vi "Phasor Convert Ratio to Amplitude Ratio & Average Lifetime.vi"(6 "Compute Amplitude Ratio":bool, 8 "error in (no error)":errorcluster, 9 "Reference Lifetime 2":dbl[unit], 10 "Reference Lifetime 1":dbl[unit], 11 "Phasor Ratio (f1)":dbl) -> (0 "error out":errorcluster, 1 "Average Lifetime":dbl[unit], 3 "Phasor/Amplitude Ratio":dbl, 4 "Average Lifetime Caption":string, 5 "Phasor Ratio Plot Name Suffix":string)   [LabVIEW 2021, in "Phasor.lvlib"]
uses:
  Phasor.lvlib
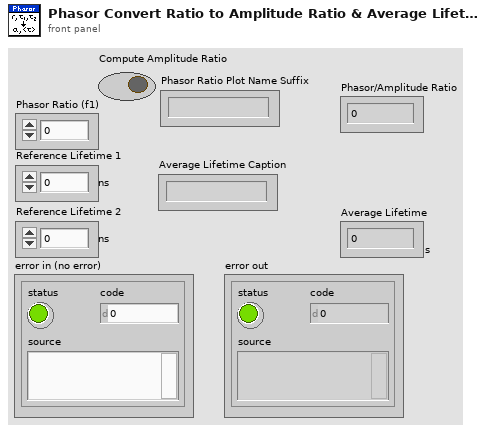
[diagram p1: front panel]
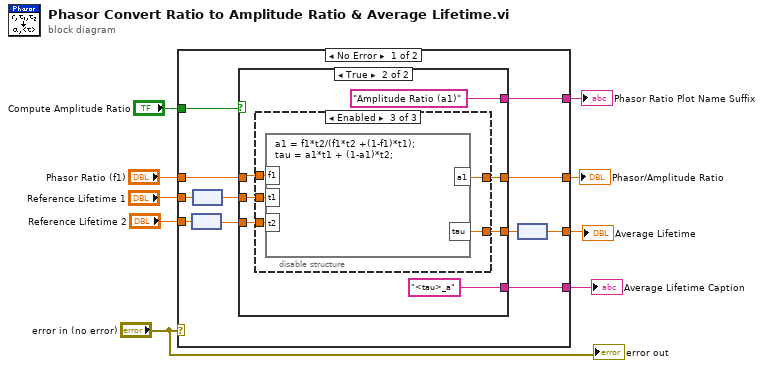
[diagram p0: block diagram]
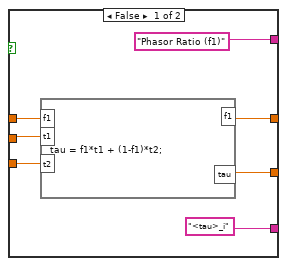
[diagram p2: hidden frame]
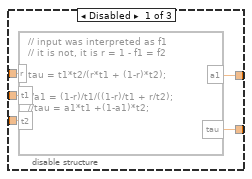
[diagram p3: hidden frame]
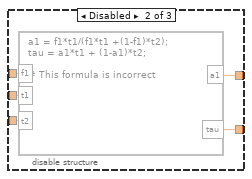
[diagram p4: hidden frame]
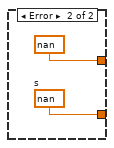
[diagram p5: hidden frame]
diagram:
  n1 = case shown="No Error" "error in (no error)" {
    tunnel: "Phasor Ratio (f1)" -> [w20 _]
    tunnel: [w19 nan ("a1")] -> w8
    tunnel: "Reference Lifetime 1" -> [w18 _]
    tunnel: "Reference Lifetime 2" -> [w16 _]
    tunnel: [w14 _] -> w5
    tunnel: [w12 w50] -> w4
    tunnel: [w11 _] -> w3
    tunnel: "Compute Amplitude Ratio" -> [w10 _]
    frame No Error {
      n2 = node(w16) -> (w15:dbl)
      n3 = node(w18) -> (w17:dbl)
      n4 = case shown="True" w10 {
        tunnel: w20 -> [w25 w31]
        tunnel: [w21 w32] -> w19
        tunnel: w17 -> [w26 w34]
        tunnel: w15 -> [w24 w33]
        tunnel: ["Phasor Ratio (f1)" ("Plot Name Suffix") "Amplitude Ratio (a1)" ("Plot Name Suffix")] -> w14
        tunnel: [w23 w29] -> w13
        tunnel: ["<tau>_i" ("Plot Name Suffix") "<tau>_a" ("Plot Name Suffix")] -> w11
        frame False {
          n5 = formula code="tau = f1*t1 + (1-f1)*t2;"("f1"=w25, "t1"=w26, "t2"=w24) -> ("tau"=w23:dbl, "f1"=w21:dbl)
        }
        frame True {
          n6 = disable-structure shown="Enabled" {
            disable-tunnel: w34 -> [w39 w44 w49]
            disable-tunnel: w33 -> [w38 w43 w48]
            disable-tunnel: [w37 w42 w47] -> w32
            disable-tunnel: w31 -> [w36 w41 w46]
            disable-tunnel: [w35 w40 w45] -> w29
            frame Disabled {
              n7 = formula code="// input was interpreted as f1\n// it is not, it is r = 1 - f1 = f2\n\ntau = t1*t2/(r*t1 + (1-r)*t2);\n\n//a1 = (1-r)/t1/((1-r)/t1 + r/t2);\n//tau = a1*t1 +(1-a1)*t2;"("r"=w36, "t1"=w39, "t2"=w38) -> ("a1"=w37:dbl, "tau"=w35:dbl)
            }
            frame Disabled {
              n8 = formula code="a1 = f1*t1/(f1*t1 +(1-f1)*t2);\ntau = a1*t1 + (1-a1)*t2;\n\n# This formula is incorrect"("f1"=w41, "t1"=w44, "t2"=w43) -> ("a1"=w42:dbl, "tau"=w40:dbl)
            }
            frame Enabled {
              n9 = formula code="a1 = f1*t2/(f1*t2 +(1-f1)*t1);\ntau = a1*t1 + (1-a1)*t2;"("f1"=w46, "t1"=w49, "t2"=w48) -> ("a1"=w47:dbl, "tau"=w45:dbl)
            }
          }
        }
      }
      n10 = node(w13) -> (w12:dbl[unit])
    }
    frame Error {
      w50 = dbl[unit] nan  # s
    }
  }
  "Phasor/Amplitude Ratio" <- w8
  "Phasor Ratio Plot Name Suffix" <- w5
  "Average Lifetime" <- w4
  "Average Lifetime Caption" <- w3
  "error out" <- "error in (no error)"
